vi "XYZStage-Standalone.vi"() -> ()   [LabVIEW 2020]
uses:
  Typedefs/XYZ channel ring.ctl
  Typedefs/Hardware Configuration settings.ctl
  Typedefs/Triggers HW config.ctl
  Typedefs/DAQmx physical channels cluster.ctl
  Control/typedefs/XYZControlConfig.ctl
  Typedefs/XY Stage config cluster.ctl
  Typedefs/Z Stage config cluster.ctl
  Typedefs/Encoder config cluster.ctl
  Typedefs/Cam VidRec HW config setup cluster.ctl
  Typedefs/Laser Power Control HW config.ctl
  Typedefs/Laser 1 config cluster.ctl
  Typedefs/PreChirper 1 config cluster.ctl
  Typedefs/Control Sys HW config cluster.ctl
  Typedefs/DAQ FPGA HW config cluster.ctl
  RIG-SPECIFIC FILES/FPGA Refs/FPGA Ref.ctl
  <vilib>/userDefined/High Color/nirio_resource_hc.ctl
  Typedefs/FPGA input type AC-DC.ctl
  Typedefs/PMT Control Voltage limits.ctl
  Typedefs/UI ctrl refs cluster.ctl
  Typedefs/HW config states enum.ctl
  Typedefs/Imaging Protocols enum.ctl
  Global Variables/General Globals.vi
  Global Variables/gl_UI Ctrl Refs.vi
  Typedefs/Set Main VI cursor.ctl
  User Interface/Windows/Position control window/Globals/Pos ctrl window globals.vi
panel:
  in  "Open Position control":bool
  out "Hardware Configuration OUT":T1={"Dev. PC"=FALSE, "Swap XY on stage"=FALSE, "No of AOD"=0, "MC Supported"=FALSE, "Axial MC"=FALSE, "Computer MAC address"="", "Externalise Triggers"=FALSE, "Trigger HW config"={"Available Device List"=0, "Device Address"=""}, "DAQmx Chan"={"Pockels AO"="", "Hard shutter AO"="", "PMT AOs"="", "Galvo AOs"="", "Power meter AI"=""}, "XYZ Stage Control Config"=enum."None", "XY stage available"=FALSE, "XY Stage"={"COM port"="", "Baudrate"=0, "Type"=""}, "Z stage available"=FALSE, "Z Stage config cluster"={"COM port"="COM7", "Baudrate"=0, "Type"=""}, "Encoder available"=FALSE, "Encoder"={"IP address"="224.0.1.103", "Port"=7000, "Wheel radius (cm)"=16.0, "Encoder Trigger"=""}, "VidRec available"=FALSE, "Cam VidRec"={"DO flag-Video record"="", "DO flag-Trial start"=""}, "Laser Power Control HW config"={"Laser Power Control"="", "Laser Power Modulation Control"=enum."NI"}, "Laser 1 available"=FALSE, "Laser 1 config cluster"={"COM port"="COM7", "Baud Rate"=0, "Type"=""}, "Prechirper 1 available"=FALSE, "Prechirper 1 config cluster"={"Type"="", "Baud Rate"=0, "COM port"="COM7"}, "Control system.FPGA available?"=FALSE, "Control Sys. HW config"={"Control system.FPGA Type"=enum."Virtex 5", "Control system.Network adapter name"="", "Control system.MAC address"="", "Control system.Ethernet Port"=0, "Control system.Ethernet Port Opened"=FALSE}, "DAQ FPGA HW Config"={"FGPA Ref"=refnum, "Target"="RIO0", "input card type"=enum."AC Card"}, "PMT Control Voltage Limits"={"Lower Limit"=0.0, "Upper Limit"=0.0}} {"Encoder"."Wheel radius (cm)" format="%#_13g"}
  in  "stop":bool
  out "Stage XYZ Position":cluster{"X":sgl, "Y":sgl, "Z":sgl} caption="Current Stage Position (µm)" {"Z" format="Z:%#_g"; "Y" format="Y:%#_g"; "X" format="X:%#_g"}
  in  "Axis":T18="All" caption="Axis to zero"
  in  "Set as Origin":bool
  in  "error in (no error)":errorcluster
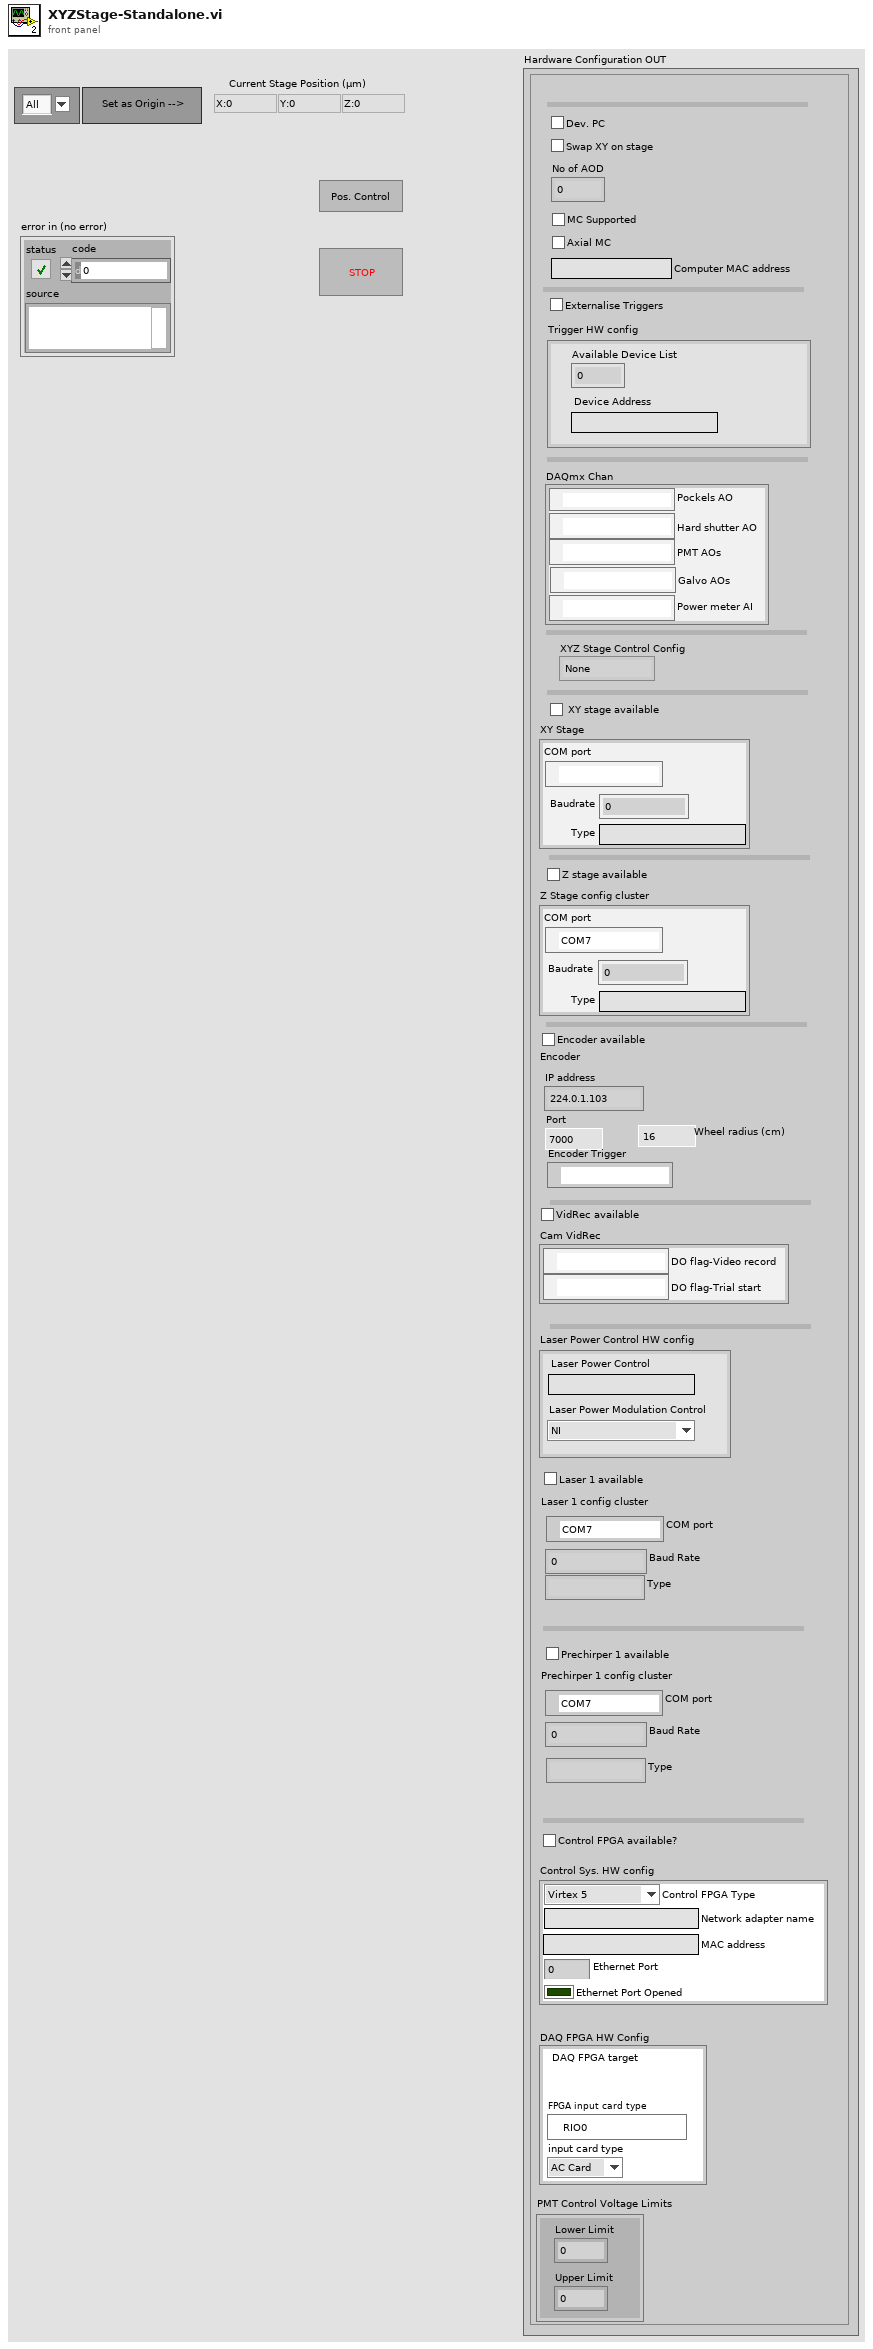
[diagram p1: front panel]
types:
  T1 = typedef "Hardware Configuration settings.ctl" = cluster{"Dev. PC":bool, "Swap XY on stage":bool, "No of AOD":u8, "MC Supported":bool, "Axial MC":bool, "Computer MAC address":string, "Externalise Triggers":bool, "Trigger HW config":T2, "DAQmx Chan":T3, "XYZ Stage Control Config":T4, "XY stage available":bool, "XY Stage":T5, "Z stage available":bool, "Z Stage config cluster":T6, "Encoder available":bool, "Encoder":T7, "VidRec available":bool, "Cam VidRec":T8, "Laser Power Control HW config":T9, "Laser 1 available":bool, "Laser 1 config cluster":T10, "Prechirper 1 available":bool, "Prechirper 1 config cluster":T11, "Control system.FPGA available?":bool, "Control Sys. HW config":T12, "DAQ FPGA HW Config":T13, "PMT Control Voltage Limits":T17}
  T2 = typedef "Triggers HW config.ctl" = cluster{"Available Device List":i32, "Device Address":string}
  T3 = typedef "DAQmx physical channels cluster.ctl" = cluster{"Pockels AO":tag, "Hard shutter AO":tag, "PMT AOs":tag, "Galvo AOs":tag, "Power meter AI":tag}
  T4 = typedef "XYZControlConfig.ctl" = enum16{"None", "XYZ", "XY-Z", "X-Y-Z", "Z"}
  T5 = typedef "XY Stage config cluster.ctl" = cluster{"COM port":refnum<visa-resource-name>, "Baudrate":i32, "Type":string}
  T6 = typedef "Z Stage config cluster.ctl" = cluster{"COM port":refnum<visa-resource-name>, "Baudrate":i32, "Type":string}
  T7 = typedef "Encoder config cluster.ctl" = cluster{"IP address":string, "Port":u16, "Wheel radius (cm)":dbl, "Encoder Trigger":tag}
  T8 = typedef "Cam VidRec HW config setup cluster.ctl" = cluster{"DO flag-Video record":tag, "DO flag-Trial start":tag}
  T9 = typedef "Laser Power Control HW config.ctl" = cluster{"Laser Power Control":string, "Laser Power Modulation Control":enum16{"NI", "FPGA"}}
  T10 = typedef "Laser 1 config cluster.ctl" = cluster{"COM port":refnum<visa-resource-name>, "Baud Rate":i32, "Type":string}
  T11 = typedef "PreChirper 1 config cluster.ctl" = cluster{"Type":string, "Baud Rate":i32, "COM port":refnum<visa-resource-name>}
  T12 = typedef "Control Sys HW config cluster.ctl" = cluster{"Control system.FPGA Type":enum16{"Virtex 5", "Virtex 7"}, "Control system.Network adapter name":string, "Control system.MAC address":string, "Control system.Ethernet Port":u32, "Control system.Ethernet Port Opened":bool}
  T13 = typedef "DAQ FPGA HW config cluster.ctl" = cluster{"FGPA Ref":T14, "Target":T15, "input card type":T16}
  T14 = typedef "FPGA Ref.ctl" = refnum<k20>
  T15 = typedef "nirio_resource_hc.ctl" = tag
  T16 = typedef "FPGA input type AC-DC.ctl" = enum16{"AC Card", "DC Card"}
  T17 = typedef "PMT Control Voltage limits.ctl" = cluster{"Lower Limit":dbl, "Upper Limit":dbl}
  T18 = typedef "XYZ channel ring.ctl" = string
  T19 = typedef "UI ctrl refs cluster.ctl" = cluster{"Top level VI path":path, "Top level VI ref":refnum<vi>, "User menu ref":refnum<k9>, "Sub Panel control":refnum<vi>, "Imaging Param Tab":refnum<vi>, "Occurrence-Start drivers":refnum<k4>, "Occurrence-Speed logging initialised":refnum<k4>, "Occurrence-XYZ stage initialised":refnum<k4>, "Exit button":refnum<vi>, "Status ind":refnum<vi>, "Set as origin":refnum<vi>, "Speed Logging":refnum<vi>, "Time Lapse":refnum<vi>, "Live Imaging":refnum<vi>, "AOL Z Stack":refnum<vi>, "Motor Z Stack":refnum<vi>, "Funct Acq button":refnum<vi>, "Hard Shutter":refnum<vi>, "Virtual Shutter":refnum<vi>, "Laser Power":refnum<vi>, "AOL Mode":refnum<vi>, "Frame Size":refnum<vi>, "Field of View":refnum<vi>, "Dwell Time":refnum<vi>, "Zoom":refnum<vi>, "AOL Z":refnum<vi>, "Objective":refnum<vi>, "Axis":refnum<vi>, "Paths & Names":refnum<vi>, "Experiment folder path (ind.)":refnum<vi>, "Last State (Ind.)":refnum<vi>, "Averages":refnum<vi>, "Angle (degrees)":refnum<vi>, "X centre":refnum<vi>, "Y centre":refnum<vi>, "Plane Mode":refnum<vi>, "# Planes":refnum<vi>, "Z Start":refnum<vi>, "Z Stop":refnum<vi>, "Z Step":refnum<vi>, "PMT 1":refnum<vi>, "PMT 2":refnum<vi>, "Stage XYZ Position":refnum<vi>, "Pockels@Z Start":refnum<vi>, "Pockels@Z Stop":refnum<vi>, "Obtain Z Start":refnum<vi>, "Obtain Z Stop":refnum<vi>, "Live stim.trig.period":refnum<vi>, "Live stim.trig.enable":refnum<vi>, "Movement Correction":refnum<vi>, "Load Reference Image":refnum<vi>, "XY Stage Move":refnum<vi>, "MovCor Cluster":refnum<vi>, "RefDAQParam":refnum<vi>, "Funct. Acq. Pockels Modulation":refnum<vi>, "Ref Laser Power":refnum<vi>, "Enable Video Recording":refnum<vi>, "Video Record-Live Imaging":refnum<vi>, "Video Record-Funct acq":refnum<vi>, "Reference Source":refnum<vi>, "AOL Z-stack Chirps Ready (ind)":refnum<vi>, "Target time between mov.cor. ref triggers (ms)":refnum<vi>, "Funct. Acq. Ref frame save":refnum<vi>, "Tracking button":refnum<vi>, "Show ref plots window":refnum<vi>, "Center freq ind (nm)":refnum<vi>, "Pickup mode (ind)":refnum<vi>, "Logging queue (ind)":refnum<vi>, "Back aperture power (ind.)":refnum<vi>, "Power after objective (ind.)":refnum<vi>, "Switch user":refnum<vi>, "Ls1 Conn. Status":refnum<vi>, "Ls1Tuning Status":refnum<vi>, "Ls1 Faults":refnum<vi>, "Ls1 Connection":refnum<vi>, "Ls1 Mode":refnum<vi>, "Ls1 POWER [mW]":refnum<vi>, "Ls1Shutter":refnum<vi>, "Ls1 Wavelength":refnum<vi>, "Ls1 Note":refnum<vi>, "Ls1 Confirm Wav":refnum<vi>, "Ls1 PreChrp Prism1":refnum<vi>, "Ls1 PreChrp Prism2":refnum<vi>, "Ls1 wav top Ind":refnum<vi>, "Ls1 power top Ind":refnum<vi>, "Ls1 Pump peak Hold":refnum<vi>, "Ls1 Status Ind":refnum<vi>, "Ls1 wav cancel":refnum<vi>, "Experiment Type":refnum<vi>, "Biology Information":refnum<vi>}
  T20 = typedef "Imaging Protocols enum.ctl" = enum16{"AOL Z-Stack", "Motor Z Stack", "Functional Acquisition", "Single Plane Acquisition", "Volume Acquisition", "Live Imaging", "Live Plane Imaging", "Live Volume Imaging"}
  T21 = typedef "HW config states enum.ctl" = enum16{"Load from file", "Save to file", "Write all", "Read all", "Write XY stage settings", "Write DAQ FPGA settings", "Write Control FPGA settings", "Write Phys Channels", "Write System Config", "Write HW Config", "Save System Config", "Save HW Config", "Clear", "Compare from file"}
  T22 = typedef "Set Main VI cursor.ctl" = enum16{"Release busy cursor", "Set busy cursor"}
  T23 = typedef "AOL_Globals.ctl" = cluster{"Imaging Protocol":T20, "Number of POI":u16, "Number of Miniscans":u16, "Number of Trials":u16, "Number of Cycles ":u64, "# Averaged Frames":u16, "Laser power (%)":u8, "Pockels (V)":dbl, "Acquisition Length (sec)":dbl, "Fill time (us)":dbl, "POI Dwell time (us)":dbl, "Miniscan Dwell time per pixel (us)":dbl, "PMT 1":dbl, "PMT 2":dbl, "Back Apperture (mA)":dbl, "Frame Size":T24, "Center Frequency":dbl, "Field of View (norm)":dbl, "DwellTime (us)":dbl, "Wavelength (nm)":dbl, "Zoom":dbl, "AOL Z":dbl, "AOL Mode":T25, "GridXY":dbl, "GridZ":dbl, "TriggerPeriod (sec)":dbl, "Number of Pixels in Miniscan":u16, "Experiment folder path":path, "X centre":dbl, "Y centre":dbl, "Angle (degrees)":dbl, "Angle Xs (degrees)":dbl, "Angle Ys (degrees)":dbl, "Plane Mode":T26, "Threshold":u16[], "Regenerate Chirps":bool, "Rectangle ROI length (pixels)":u16, "Rectangle ROI height (pixels)":u16, "AOD fill":u16, "StartupDelay":i32, "Samples Wait after Trigger":u16, "Slip Cycle":u32, "Add Cycle":bool, "Functional Mode":T27, "Z Start":dbl, "Z Stop":dbl, "# Planes":i32, "Field of View [um] ":dbl}
  T24 = typedef "Frame Size.ctl" = u16
  T25 = typedef "AOL modes.ctl" = enum16{"Raster", "Structural", "Pointing", "Mini Scan", "Alignment"}
  T26 = typedef "Plane Mode.ctl" = u16
  T27 = typedef "Functional Mode.ctl" = enum16{"Point", "Line", "Patch", "Plane", "Volume"}
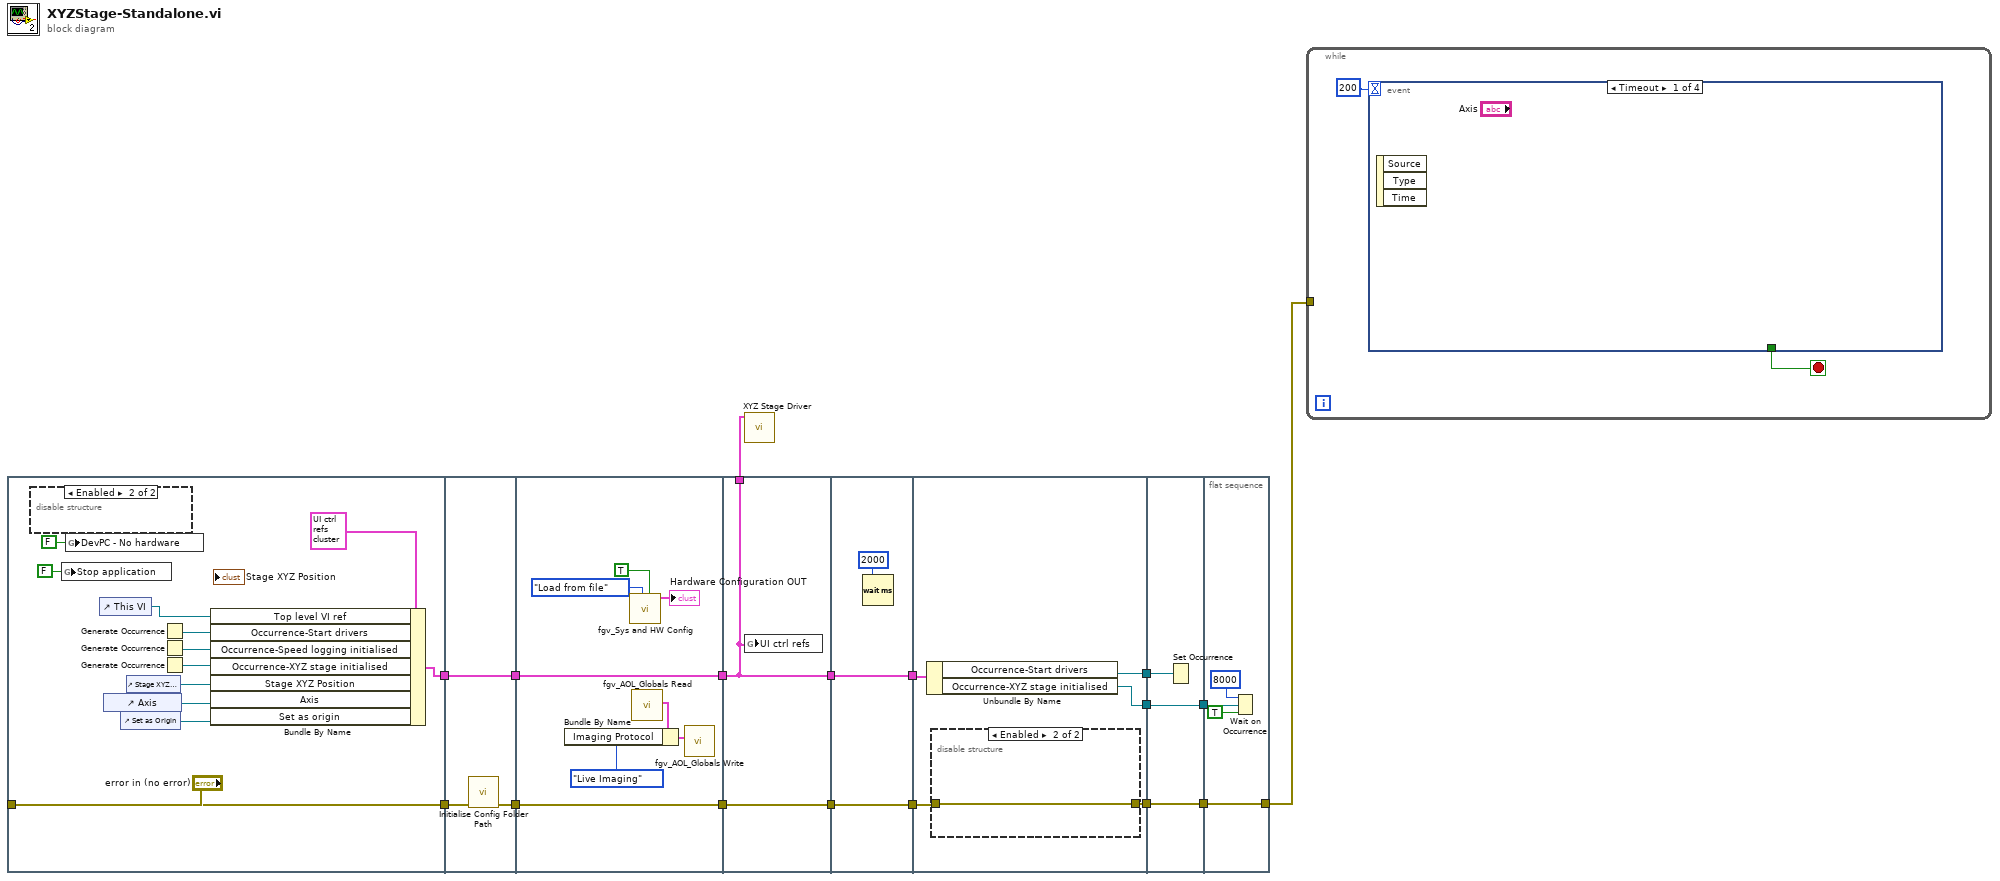
[diagram p0: block diagram]
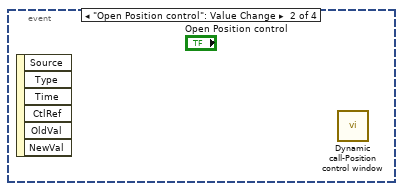
[diagram p2: hidden frame]
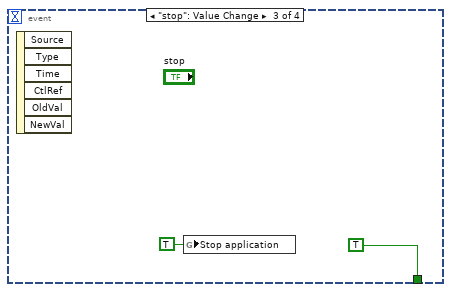
[diagram p3: hidden frame]
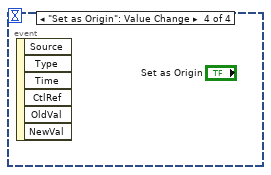
[diagram p4: hidden frame]
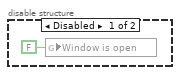
[diagram p5: hidden frame]
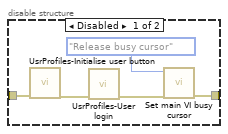
[diagram p6: hidden frame]
diagram:
  n1 = flat-sequence {
    tunnel: "error in (no error)" -> [w23]
    tunnel: [w23] -> w4
    tunnel: [w21] -> w2
    tunnel: w4 -> [w33]
    tunnel: [w32] -> w3
    tunnel: w2 -> [w34]
    tunnel: [w34] -> w1
    tunnel: w3 -> [w42]
    tunnel: [w42] -> w9
    tunnel: w1 -> [w41]
    tunnel: [w41] -> w7
    tunnel: w9 -> [w44]
    tunnel: [w44] -> w8
    tunnel: w7 -> [w43]
    tunnel: [w43] -> w6
    tunnel: [w43] -> w5
    tunnel: w8 -> [w47]
    tunnel: [w47] -> w11
    tunnel: w6 -> [w46]
    tunnel: [w46] -> w10
    tunnel: w11 -> [w48]
    tunnel: w10 -> [w49]
    tunnel: [w50] -> w17
    tunnel: [w52] -> w16
    tunnel: [w51] -> w13
    tunnel: w17 -> [w61]
    tunnel: w16 -> [w60]
    tunnel: [w61] -> w15
    tunnel: [w59] -> w14
    tunnel: w13 -> [w59]
    tunnel: [w65] -> w12
    tunnel: w15 -> [w65]
    tunnel: w14 -> [w64]
    frame #0 {
      n2 = disable-structure shown="Enabled" {
        frame Disabled {
          n3 = global write "Pos ctrl window globals.vi" "Window is open"(FALSE ("Window is open")) -> ()
        }
        frame Enabled {
        }
      }
      n4 = global write "General Globals.vi" "Stop application"(FALSE ("Stop application")) -> ()
      n5 = global write "General Globals.vi" "DevPC - No hardware"(FALSE ("DevPC - No hardware")) -> ()
      n6 = control-ref of="This VI"() -> (w19:refnum<vi>)
      n7 = control-ref of="Axis"() -> (w25:refnum<vi>)
      n8 = control-ref of="Set as Origin"() -> (w24:refnum<vi>)
      n9 = control-ref of="Stage XYZ Position"() -> (w26:refnum<vi>)
      n10 = Generate Occurrence() -> (w29:refnum<k4>)
      n11 = Generate Occurrence() -> (w28:refnum<k4>)
      n12 = Generate Occurrence() -> (w27:refnum<k4>)
      n13 = Bundle By Name(cluster=T19 {"Top level VI path"=path "", "Top level VI ref"=refnum, "User menu ref"=refnum, "Sub Panel control"=refnum, "Imaging Param Tab"=refnum, "Occurrence-Start drivers"=refnum, "Occurrence-Speed logging initialised"=refnum, "Occurrence-XYZ stage initialised"=refnum, "Exit button"=refnum, "Status ind"=refnum, "Set as origin"=refnum, "Speed Logging"=refnum, "Time Lapse"=refnum, "Live Imaging"=refnum, "AOL Z Stack"=refnum, "Motor Z Stack"=refnum, "Funct Acq button"=refnum, "Hard Shutter"=refnum, "Virtual Shutter"=refnum, "Laser Power"=refnum, "AOL Mode"=refnum, "Frame Size"=refnum, "Field of View"=refnum, "Dwell Time"=refnum, "Zoom"=refnum, "AOL Z"=refnum, "Objective"=refnum, "Axis"=refnum, "Paths & Names"=refnum, "Experiment folder path (ind.)"=refnum, "Last State (Ind.)"=refnum, "Averages"=refnum, "Angle (degrees)"=refnum, "X centre"=refnum, "Y centre"=refnum, "Plane Mode"=refnum, "# Planes"=refnum, "Z Start"=refnum, "Z Stop"=refnum, "Z Step"=refnum, "PMT 1"=refnum, "PMT 2"=refnum, "Stage XYZ Position"=refnum, "Pockels@Z Start"=refnum, "Pockels@Z Stop"=refnum, "Obtain Z Start"=refnum, "Obtain Z Stop"=refnum, "Live stim.trig.period"=refnum, "Live stim.trig.enable"=refnum, "Movement Correction"=refnum, "Load Reference Image"=refnum, "XY Stage Move"=refnum, "MovCor Cluster"=refnum, "RefDAQParam"=refnum, "Funct. Acq. Pockels Modulation"=refnum, "Ref Laser Power"=refnum, "Enable Video Recording"=refnum, "Video Record-Live Imaging"=refnum, "Video Record-Funct acq"=refnum, "Reference Source"=refnum, "AOL Z-stack Chirps Ready (ind)"=refnum, "Target time between mov.cor. ref triggers (ms)"=refnum, "Funct. Acq. Ref frame save"=refnum, "Tracking button"=refnum, "Show ref plots window"=refnum, "Center freq ind (nm)"=refnum, "Pickup mode (ind)"=refnum, "Logging queue (ind)"=refnum, "Back aperture power (ind.)"=refnum, "Power after objective (ind.)"=refnum, "Switch user"=refnum, "Ls1 Conn. Status"=refnum, "Ls1Tuning Status"=refnum, "Ls1 Faults"=refnum, "Ls1 Connection"=refnum, "Ls1 Mode"=refnum, "Ls1 POWER [mW]"=refnum, "Ls1Shutter"=refnum, "Ls1 Wavelength"=refnum, "Ls1 Note"=refnum, "Ls1 Confirm Wav"=refnum, "Ls1 PreChrp Prism1"=refnum, "Ls1 PreChrp Prism2"=refnum, "Ls1 wav top Ind"=refnum, "Ls1 power top Ind"=refnum, "Ls1 Pump peak Hold"=refnum, "Ls1 Status Ind"=refnum, "Ls1 wav cancel"=refnum, "Experiment Type"=refnum, "Biology Information"=refnum} ("output cluster"), "Top level VI ref"=w19, "Occurrence-Start drivers"=w29, "Occurrence-Speed logging initialised"=w28, "Occurrence-XYZ stage initialised"=w27, "Stage XYZ Position"=w26, "Axis"=w25, "Set as origin"=w24) -> (w21:T19)
    }
    frame #1 {
      n14 = call "Initialise Config Folder Path.vi"("error in (no error)"=w33) -> ("error out"=w32:errorcluster)  [unwired: 8 in, 2 out]
    }
    frame #2 {
      n15 = call "fgv_Sys and HW Config.vi"("Standalone viewer initialisation?"=TRUE, "Function"=HW_config_states_enum."Load from file") -> ("Hardware Configuration OUT"=→"Hardware Configuration OUT":T1)  [unwired: 7 in, 2 out]
      n16 = call "fgv_AOL_Globals Read.vi"() -> ("AOL_Globals"=w37:T23)  [unwired: 9 in, 2 out]
      n17 = Bundle By Name(cluster=w37, "Imaging Protocol"=Imaging_Protocols_enum."Live Imaging") -> (w36:T23)
      n18 = call "fgv_AOL_Globals Write.vi"("AOL_Globals"=w36) -> ()  [unwired: 10 in, 1 out]
    }
    frame #3 {
      n19 = global write "gl_UI Ctrl Refs.vi" "UI ctrl refs"(w43) -> ()
    }
    frame #4 {
      n20 = Wait (ms)(milliseconds to wait=u32 2000) -> ()  [unwired: 1 out]
    }
    frame #5 {
      n21 = Unbundle By Name(w49) -> ("Occurrence-Start drivers"=w52:refnum<k4>, "Occurrence-XYZ stage initialised"=w51:refnum<k4>)
      n22 = disable-structure shown="Enabled" {
        disable-tunnel: w48 -> [w57 w58]
        disable-tunnel: [w53 w58] -> w50
        frame Disabled {
          n23 = call "UsrProfiles-Initialise user button.vi"("error in (no error)"=w57) -> ("error out"=w56:errorcluster)  [unwired: 10 in]
          n24 = call "UsrProfiles-User login.vi"("error in (no error)"=w56) -> ("error out"=w54:errorcluster)  [unwired: 10 in]
          n25 = call "Set main VI busy cursor.vi"("error in (no error)"=w54, "Main VI's cursor"=Set_Main_VI_cursor."Release busy cursor") -> ("error out"=w53:errorcluster)  [unwired: 9 in]
        }
        frame Enabled {
        }
      }
    }
    frame #6 {
      n26 = Set Occurrence(w60) -> ()
    }
    frame #7 {
      n27 = Wait on Occurrence(1:TRUE ("ignore previous (T)"), 2:w64, 3:8000 ("ms timeout (-1)")) -> ()  [unwired: 1 out]
    }
  }
  n28 = call "XYZ Stage Driver.vi"("UI elements cluster"=w5) -> ()  [unwired: 10 in, 1 out]
  n29 = while {
    tunnel: w12 -> [_]
    stop <- w66 stop-if-true
    n30 = event shown="[0] Timeout" {
      selector: _ -> [_ _ _ _]
      dyn-events: _ -> [_ _ _ _]
      timeout: 200 -> [_ _ _ _]
      tunnel: [_ _ TRUE _] -> w66
      event Timeout {
        n31 = event-data() -> ()  [unwired: 1 in, 3 out]
      }
      event "Open Position control": Value Change {
        n32 = event-data() -> ()  [unwired: 1 in, 6 out]
        n33 = call "Dynamic call-Position control window.vi"() -> ()  [unwired: 11 in, 1 out]
      }
      event "stop": Value Change {
        n34 = event-data() -> ()  [unwired: 1 in, 6 out]
        n35 = global write "General Globals.vi" "Stop application"(TRUE ("Stop application")) -> ()
      }
      event "Set as Origin": Value Change {
        n36 = event-data() -> ()  [unwired: 1 in, 6 out]
      }
    }
  }
